vi "ReadAll.vi"(8 "error in (no error)":errorcluster, 11 "Class4 in":refnum<class "Class4.lvclass">) -> (0 "error out":errorcluster, 1 "someNumber":dbl, 2 "anotherNumber":dbl, 3 "Class4 out":refnum<class "Class4.lvclass">, 4 "myBool":bool)   [LabVIEW 2020, in "Class4.lvclass"]
doc: "GCraftsman JSON Object Serialization Toolkit\nwww.GCraftsman.com\nCopyright (c) 2017, GCraftsman"
uses:
  Class4.lvclass
  Class4.lvclass/Class4.ctl
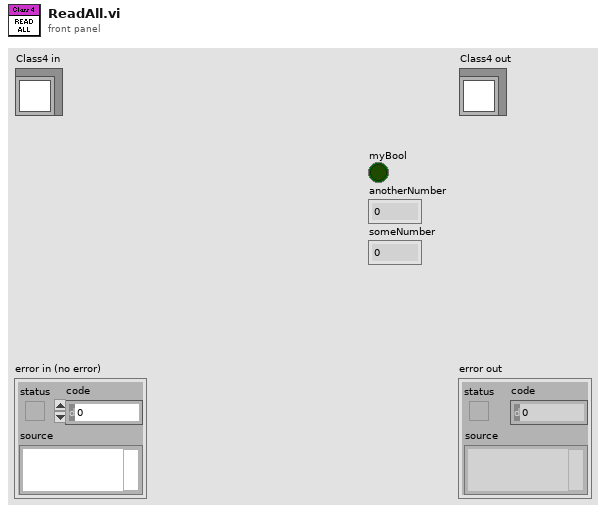
[diagram p1: front panel]
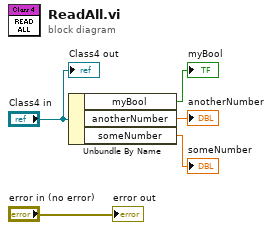
[diagram p0: block diagram]
diagram:
  n1 = Unbundle By Name("Class4 in") -> ("myBool"=→"myBool":bool, "anotherNumber"=→"anotherNumber":dbl, "someNumber"=→"someNumber":dbl)
  "error out" <- "error in (no error)"
  "Class4 out" <- "Class4 in"
